vi "闹钟（多次任意）.vi"(5 "设置时间":timestamp[](array[timestamp]), 7 "启用":bool=TRUE) -> (6 "时间到脉冲":bool, 8 "当前时间":timestamp)   [LabVIEW 2012]
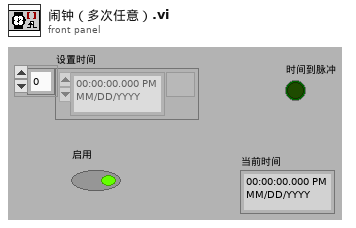
[diagram p1: front panel]
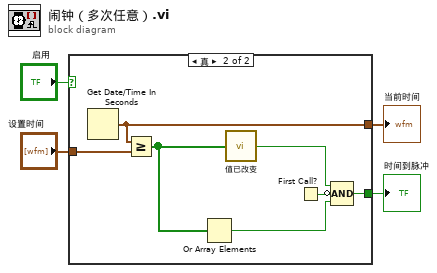
[diagram p0: block diagram]
diagram:
  n1 = case shown="真" "启用" {
    tunnel: "设置时间" -> [_ w9]
    tunnel: [_ w11] -> w2
    tunnel: [_ w5] -> w1
    frame False {
    }
    frame True {
      n2 = Get Date/Time In Seconds() -> (seconds since 1Jan1904=w5:timestamp)
      n3 = Greater Or Equal?(x=w5, y=w9) -> (x >= y?=w7:bool[])
      n4 = Or Array Elements(Boolean array=w7) -> (logical OR=w6:bool)
      n5 = call-poly "值已改变.vi"("输入数据"=w7) -> ("已更改"=w8:bool)  [unwired: 3 in]
      n6 = First Call?() -> (First Call?: T/F=w10:bool)
      n7 = Compound Arithmetic op=AND(w8, invert w10, w6) -> (w11:bool)
    }
  }
  "时间到脉冲" <- w2
  "当前时间" <- w1
